vi "Format Log AO Data.vi"(6 "Sweeping?":bool, 8 "error in (no error)":errorcluster, 10 "waveform":waveform(dbl)[](array[waveform]), 11 "Instrument.Lockin in":refnum<class "Instrument.Lockin.lvclass">) -> (0 "error out":errorcluster, 1 "Log Data":T1[](array[typedef]), 2 "Log Paths":string, 3 "Instrument.Lockin out":refnum<class "Instrument.Lockin.lvclass">, 4 "Times":timestamp[](array[timestamp]))   [LabVIEW 2019, in "Instrument.Lockin.lvlib" / "Instrument.Lockin.lvclass"]
uses:
  Instrument.Lockin.lvclass
  Typedefs/Lockin.LogSweepAOAI--Cluster.ctl
  Instrument.Lockin.lvclass/Instrument.Lockin.ctl
  Instrument.DAQ/Instrument.DAQ.lvclass
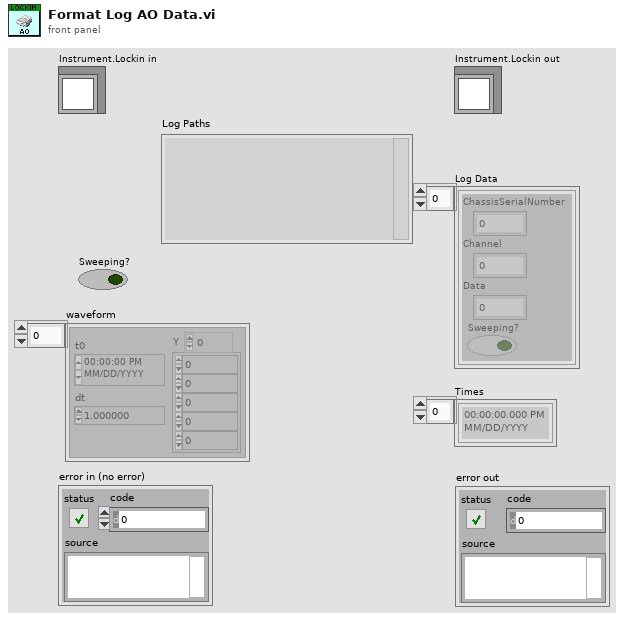
[diagram p1: front panel]
types:
  T1 = typedef "Instrument.Lockin.lvlib/Instrument.Lockin.lvclass/Lockin.LogSweepAOAI--Cluster.ctl" = cluster{"ChassisSerialNumber":u32, "Channel":i32, "Data":dbl, "Sweeping?":bool}
  T2 = typedef "Instrument.Lockin.lvlib/Instrument.DAQ.lvclass/DeviceInfo--Cluster.ctl" = cluster{"DeviceName":string, "DevIsSimulated":bool, "DeviceSerialNumber":u32, "ProductType":string, "ProductCategory":i32, "ProductNumber":u32, "ChassisNumber":u32, "SlotNumber":u32, "ChassisName":string, "ChassisSerialNumber":u32}
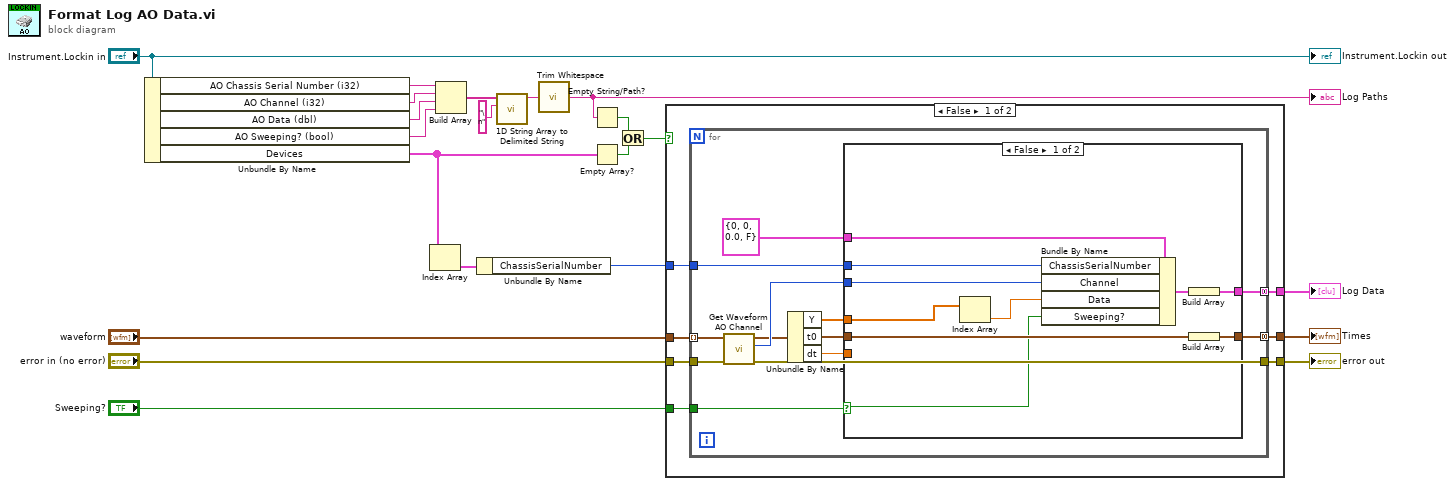
[diagram p0: block diagram]
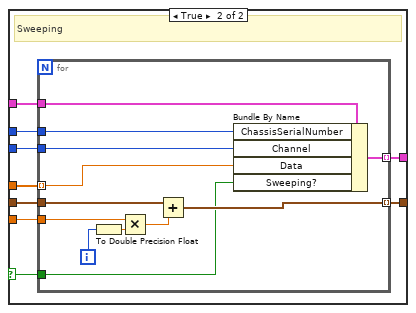
[diagram p2: hidden frame]
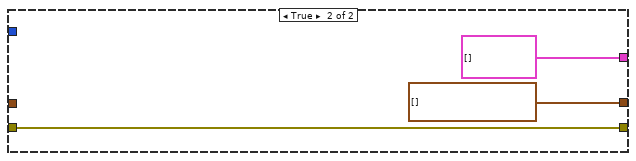
[diagram p3: hidden frame]
diagram:
  n1 = Unbundle By Name("Instrument.Lockin in") -> ("AO Chassis Serial Number (i32)"=w16:string, "AO Channel (i32)"=w1:string, "AO Data (dbl)"=w2:string, "AO Sweeping? (bool)"=w17:string, "Devices"=w3:T2[])
  n2 = Index Array(array=w3) -> (element=w12:T2)  [unwired: 1 in]
  n3 = Build Array(w16, w1, w2, w17) -> (w15:string[])
  n4 = Unbundle By Name(w12) -> ("ChassisSerialNumber"=w11:u32)
  n5 = call <vilib>:"1D String Array to Delimited String.vi"("delimiter"="\n", "string array"=w15) -> ("delimited string"=w5:string)  [unwired: 9 in]
  n6 = call <vilib>:"Trim Whitespace.vi"("string"=w5) -> ("trimmed string"=w4:string)  [unwired: 1 in]
  "Log Paths" <- w4
  n7 = Empty String/Path?(string/path=w4) -> (empty?=w7:bool)
  n8 = Empty Array?(array=w3) -> (empty?=w8:bool)
  n9 = Or(x=w7, y=w8) -> (x .or. y?=w6:bool)
  n10 = case shown="False" w6 {
    tunnel: [w28 timestamp[] []] -> w21
    tunnel: [w27 T1[] []] -> w20
    tunnel: "waveform" -> [w26 _]
    tunnel: "Sweeping?" -> [w25 _]
    tunnel: "error in (no error)" -> [w24 w73]
    tunnel: w11 -> [w23 _]
    tunnel: [w22 w73] -> w10
    frame False {
      n11 = for {
        tunnel: [w41] -> w28 mode=concatenating
        tunnel: [w40] -> w27 mode=concatenating
        tunnel: w23 -> [w39]
        tunnel: w26 -> [w32] mode=indexing
        tunnel: w25 -> [w35]
        tunnel: w24 -> [w30]
        tunnel: [w29] -> w22
        n12 = call "Get Waveform AO Channel.vi"("error in (no error)"=w30, "Reference in"=w32) -> ("error out"=w29:errorcluster, "AO Channel"=w34:i32, "Reference out"=w33:waveform(dbl))  [unwired: 7 in]
        n13 = Unbundle By Name(w33) -> ("Y"=w38:dbl[], "t0"=w36:timestamp, "dt"=w37:dbl)
        n14 = case shown="False" w35 {
          selector: w35 -> [w42 w54]
          tunnel: [w47 w60] -> w41
          tunnel: [w49 w59] -> w40
          tunnel: w39 -> [w48 w58]
          tunnel: w38 -> [w44 w57]
          tunnel: w37 -> [_ w56]
          tunnel: w36 -> [w46 w55]
          tunnel: w34 -> [w45 w53]
          tunnel: T1 {"ChassisSerialNumber"=0, "Channel"=0, "Data"=0.0, "Sweeping?"=FALSE} ("cluster") -> [w51 w52]
          frame False {
            n15 = Index Array(array=w44) -> (element=w43:dbl)  [unwired: 1 in]
            n16 = Bundle By Name(cluster=w51, "ChassisSerialNumber"=w48, "Channel"=w45, "Data"=w43, "Sweeping?"=w42) -> (w50:T1)
            n17 = Build Array(w50) -> (w49:T1[])
            n18 = Build Array(w46) -> (w47:timestamp[])
          }
          frame True {
            # "Sweeping"
            n19 = for {
              tunnel: w55 -> [w68]
              tunnel: w56 -> [w72]
              tunnel: [w67] -> w60 mode=indexing
              tunnel: w57 -> [w66] mode=indexing
              tunnel: w58 -> [w65]
              tunnel: w53 -> [w64]
              tunnel: w54 -> [w63]
              tunnel: [w62] -> w59 mode=indexing
              tunnel: w52 -> [w61]
              i -> [w71]
              n20 = To Double Precision Float(number=w71) -> (double precision float=w70:dbl)
              n21 = Multiply(x=w72, y=w70) -> (x*y=w69:dbl)
              n22 = Add(x=w68, y=w69) -> (x+y=w67:timestamp)
              n23 = Bundle By Name(cluster=w61, "ChassisSerialNumber"=w65, "Channel"=w64, "Data"=w66, "Sweeping?"=w63) -> (w62:T1)
            }
          }
        }
      }
    }
    frame True {
    }
  }
  "Times" <- w21
  "Log Data" <- w20
  "error out" <- w10
  "Instrument.Lockin out" <- "Instrument.Lockin in"
